vi "Result.Measurement, Count Fail and Errors.vi"(11 "MeasData":T1[](array[typedef]) {"Status" items=["LOG", "PASS", "FAIL", "ERROR"]}) -> (2 "Error Cnt":i32, 3 "Fail Cnt":i32)   [LabVIEW 2019]
uses:
  Result.Measurement Item.ctl
  Result.Measurement and Attribute Item Status.ctl
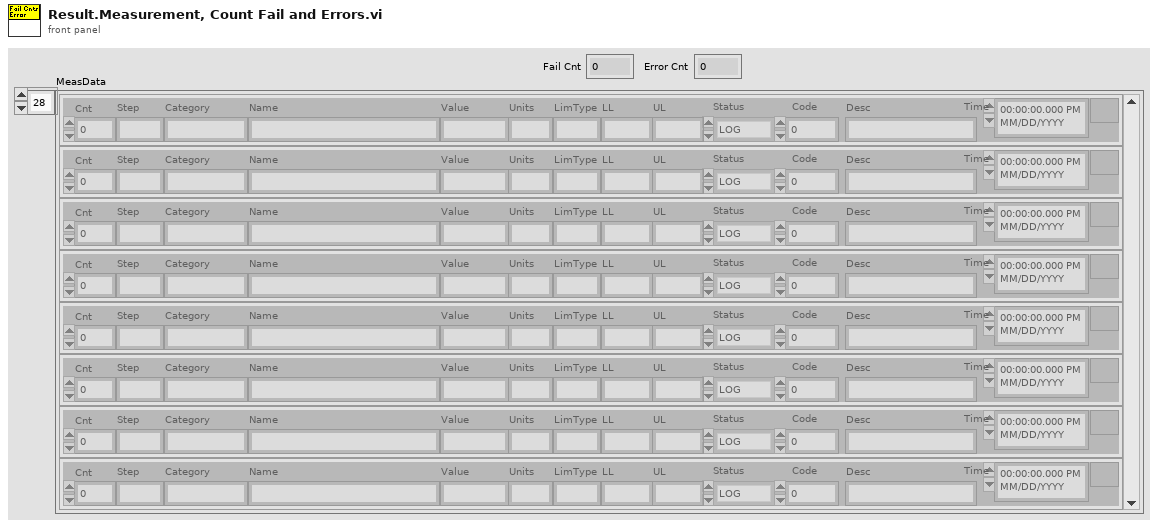
[diagram p1: front panel]
types:
  T1 = typedef "Result.Measurement Item.ctl" = cluster{"Cnt":i32, "Step":string, "Category":string, "Name":string, "Value":string, "Units":string, "LimType":string, "LL":string, "UL":string, "Status":T2, "Code":i32, "Desc":string, "Time":timestamp}
  T2 = typedef "Result.Measurement and Attribute Item Status.ctl" = i32
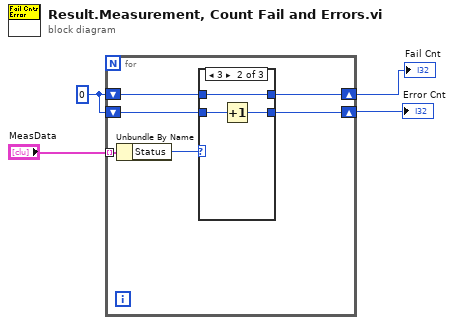
[diagram p0: block diagram]
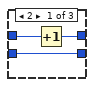
[diagram p2: hidden frame]
diagram:
  w3 = 0
  n1 = for {
    tunnel: "MeasData" -> [w10] mode=indexing
    shift-right: [w6] -> w1
    shift-left: w3 -> [w8]
    shift-right: [w5] -> w2
    shift-left: w3 -> [w7]
    n2 = Unbundle By Name(w10) -> ("Status"=w9:T2)
    n3 = case shown="3" w9 {
      tunnel: w8 -> [w11 w15 w18]
      tunnel: w7 -> [w12 w16 w17]
      tunnel: [w13 w15 w18] -> w6
      tunnel: [w12 w14 w17] -> w5
      frame 2 {
        n4 = Increment(x=w11) -> (x+1=w13:i32)
      }
      frame 3 {
        n5 = Increment(x=w16) -> (x+1=w14:i32)
      }
      frame Default {
      }
    }
  }
  "Fail Cnt" <- w1
  "Error Cnt" <- w2
